vi "Agilent VNA Read Number of Available Channels.vi"(7 "Agilent VNA":T1, 8 "error in (no error)":errorcluster, 11 "VISA Resource Name":refnum<visa-resource-name>) -> (0 "error out":errorcluster, 2 "Number of Channels":i8, 3 "dup VISA Resource Name":refnum<visa-resource-name>)   [LabVIEW 2011]
doc: "This VI for the HP 8753 is used to read the sweep type.\n\n0 LINEAR FREQ\n1 LOG FREQ\n2 LIST FREQ\n3 CW TIME\n4 POWER SWEEP"
uses:
  TypeDefs/Agilent VNA Instrument Info.ctl
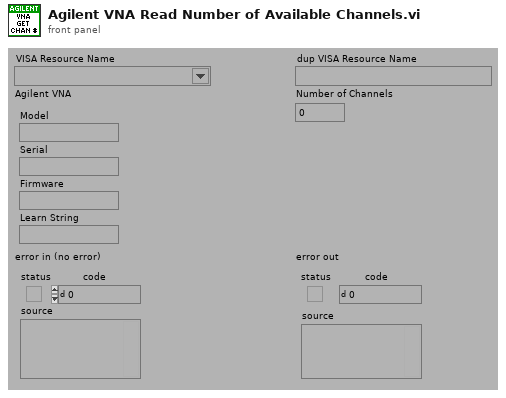
[diagram p1: front panel]
types:
  T1 = typedef "Agilent VNA Instrument Info.ctl" = cluster{"Model":string, "Serial":string, "Firmware":string, "Learn String":string}
  T2 = typedef "Agilent VNA Model.ctl" = enum16{"Not Supported", "8510X", "8719X", "8720X", "8722X", "8753X", "ENA", "PNA", "Field Fox"}
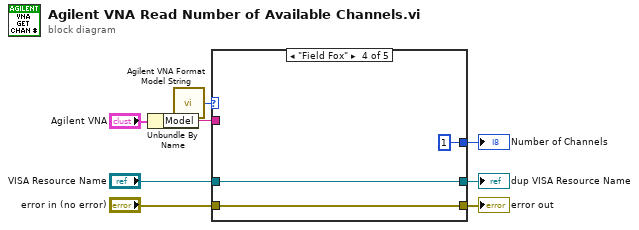
[diagram p0: block diagram]
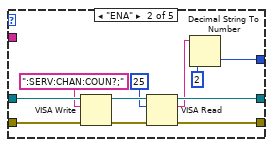
[diagram p3: hidden frame]
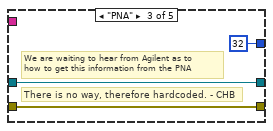
[diagram p4: hidden frame]
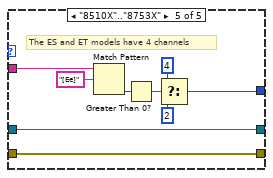
[diagram p5: hidden frame]
diagram:
  n1 = Unbundle By Name("Agilent VNA") -> ("Model"=w1:string)
  n2 = call "Agilent VNA Format Model String.vi"("Model"=w1) -> ("Model"=w3:T2)
  n3 = case shown="\"Field Fox\"" w3 {
    tunnel: "VISA Resource Name" -> [w10 w17 w23 w26 w35]
    tunnel: "error in (no error)" -> [w9 w21 w22 w25 w36]
    tunnel: [w9 w20 w22 w25 w36] -> w7
    tunnel: [_ w12 i8 32 ("Number of Channels") i8 1 ("Number of Channels") w28] -> w6
    tunnel: [w10 w15 w23 w26 w35] -> w4
    tunnel: w1 -> [_ _ _ _ w34]
    frame "Not Supported" {
    }
    frame "ENA" {
      n4 = VISA Write(VISA resource name=w17, write buffer=":SERV:CHAN:COUN?;", error in (no error)=w21) -> (VISA resource name out=w18:refnum<visa-resource-name>, error out=w19:errorcluster)  [unwired: 1 out]
      n5 = VISA Read(VISA resource name=w18, byte count=u32 25, error in (no error)=w19) -> (VISA resource name out=w15:refnum<visa-resource-name>, read buffer=w14:string, error out=w20:errorcluster)  [unwired: 1 out]
      n6 = Decimal String To Number(string=w14, default (0L)=i8 2 ("Number of Channels")) -> (number=w12:i8)  [unwired: 2 out]
    }
    frame "PNA" {
      # "There is no way, therefore hardcoded. - CHB"
      # "We are waiting to hear from Agilent as to\nhow to get this information from the PNA"
    }
    frame "Field Fox" {
    }
    frame "8510X".."8753X" {
      # "The ES and ET models have 4 channels"
      n7 = Match Pattern(string=w34, regular expression="[Ee]") -> (offset past match=w32:i32)  [unwired: 4 out]
      n8 = Greater Than 0?(x=w32) -> (x > 0?=w31:bool)
      n9 = Select(t=i8 4, s=w31, f=i8 2) -> (s? t:f=w28:i8)
    }
  }
  "Number of Channels" <- w6
  "dup VISA Resource Name" <- w4
  "error out" <- w7
